vi "Start.vi"(8 "error in (no error)":errorcluster, 11 "Stream":refnum<data-value>) -> (0 "error out":errorcluster, 3 "Stream (duplicate)":refnum<data-value>)   [LabVIEW 2020, in "g_ar_toolkit.capture.lvlib" / "CameraStream.lvclass"]
uses:
  CameraStream.lvclass
  CameraStream.lvclass/CameraStream.ctl
  bin/g_ar_toolkit.1.32.dll
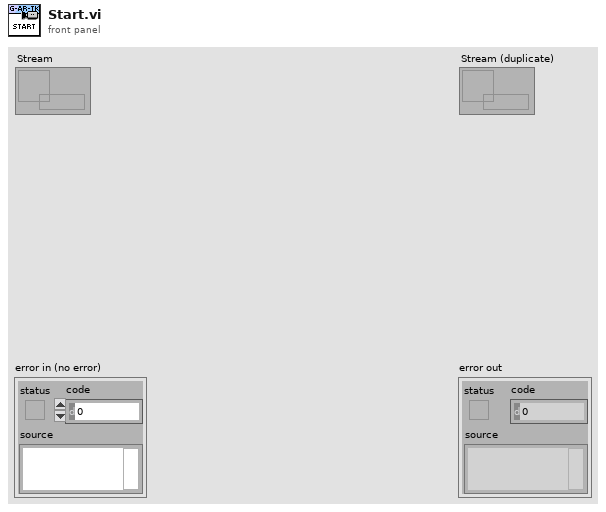
[diagram p1: front panel]
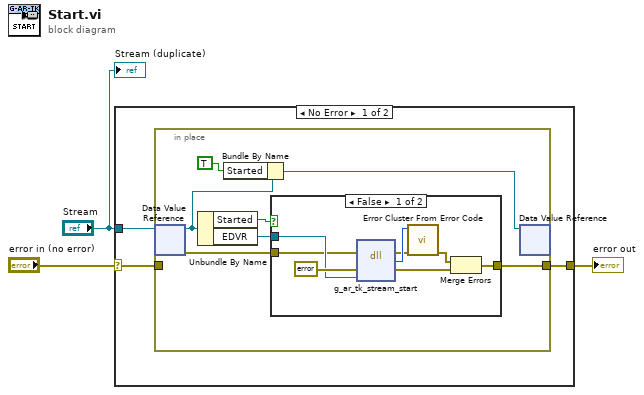
[diagram p0: block diagram]
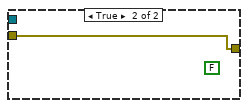
[diagram p2: hidden frame]
diagram:
  n1 = case shown="No Error" "error in (no error)" {
    selector: "error in (no error)" -> [w6 w23]
    tunnel: [w5 w23] -> w2
    tunnel: "Stream" -> [w4 _]
    frame No Error {
      n2 = in-place {
        in-place-border: w6 -> [_]
        in-place-border: [w13] -> w5
        n3 = in-place-dvr #1(w4) -> (w10:refnum<class "CameraStream.lvclass">, w11:errorcluster)
        n4 = Unbundle By Name(w10) -> ("Started"=w9:bool, "EDVR"=w12:refnum<data-value>)
        n5 = Bundle By Name(cluster=w10, "Started"=TRUE) -> (w8:refnum<class "CameraStream.lvclass">)
        n6 = case shown="False" w9 {
          tunnel: [w17 w22] -> w13
          tunnel: w12 -> [w15 _]
          tunnel: w11 -> [w14 w22]
          frame False {
            n7 = dll-call lib="C:/serenial/libraries/g-augmented-reality-toolkit/LabVIEW/bin/g_ar_toolkit.1.*.*" fn="g_ar_tk_stream_start"(error in=w14, "error_cluster"=errorcluster {"status"=FALSE, "code"=0, "source"=""} ("error constant"), "EDVR_strm"=w15) -> (error out=w20:errorcluster, "MgErr"=w21:i32, "error_cluster"=w18:errorcluster)  [unwired: 3 in, 1 out]
            n8 = call <vilib>:"Error Cluster From Error Code.vi"("error in (no error)"=w20, "error code (0)"=w21) -> ("error out"=w19:errorcluster)  [unwired: 7 in]
            n9 = Merge Errors(w19, w18) -> (w17:errorcluster)
          }
          frame True {
            (unwired) FALSE ("result")
          }
        }
        n10 = in-place-dvr #1(w8) -> ()  [unwired: 2 out]
      }
    }
    frame Error {
    }
  }
  "error out" <- w2
  "Stream (duplicate)" <- "Stream"
